vi "Delay.set.vi"(8 "error in (no error)":errorcluster, 10 "Delay (s)":dbl, 11 "comic_crawler in":refnum<class "comic_crawler.lvclass">) -> (0 "error out":errorcluster, 3 "comic_crawler out":refnum<class "comic_crawler.lvclass">)   [LabVIEW 2024, in "comic_crawler.lvclass"]
uses:
  comic_crawler.lvclass
  private/daemon.states--enum.ctl
  comic_crawler.lvclass/comic_crawler.ctl
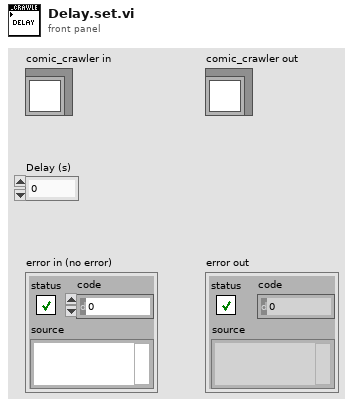
[diagram p1: front panel]
types:
  T1 = typedef "comic_crawler.lvclass/daemon.states--enum.ctl" = enum16{"start search", "idle", "set timer", "running", "stop search", "wait", "set delay", "shut down"}
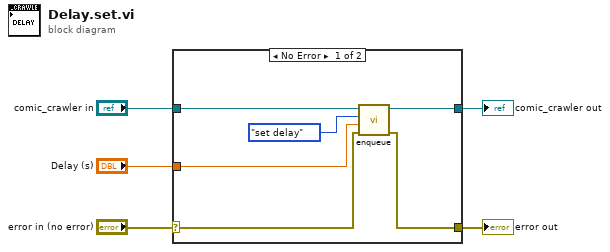
[diagram p0: block diagram]
diagram:
  n1 = case shown="No Error" "error in (no error)" {
    selector: "error in (no error)" -> [w9 w13]
    tunnel: [w8 w13] -> w4
    tunnel: [w11 w12] -> w2
    tunnel: "comic_crawler in" -> [w10 w12]
    tunnel: "Delay (s)" -> [w6 _]
    frame No Error {
      n2 = call "enqueue.vi"("error in (no error)"=w9, "data"=w6, "cmd"=daemon.states--enum."set delay", "comic_crawler in"=w10) -> ("error out"=w8:errorcluster, "comic_crawler out"=w11:refnum<class "comic_crawler.lvclass">)  [unwired: 6 in]
    }
    frame Error {
    }
  }
  "error out" <- w4
  "comic_crawler out" <- w2
